vi "SLL DE Get the order of Virtual Channels.vi"(8 "error in (no error)":errorcluster, 9 "Virtial Channels Info":string[](array[string]), 10 "Number of elements":i32[](array[numeric]), 11 "Channel Names":string[][](array[string])) -> (0 "error out":errorcluster, 3 "Channel Order":i32[](array[numeric]))   [LabVIEW 2013]
doc: "Copyright © 2005, Soliton Technologies.\nAll rights reserved."
uses:
  Instance           1 48Saved   SLL DE Get the order of Virtual Channels .vi
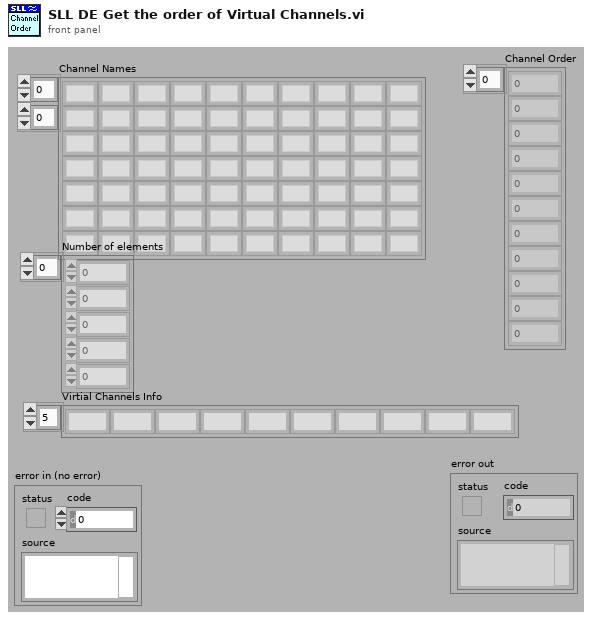
[diagram p1: front panel]
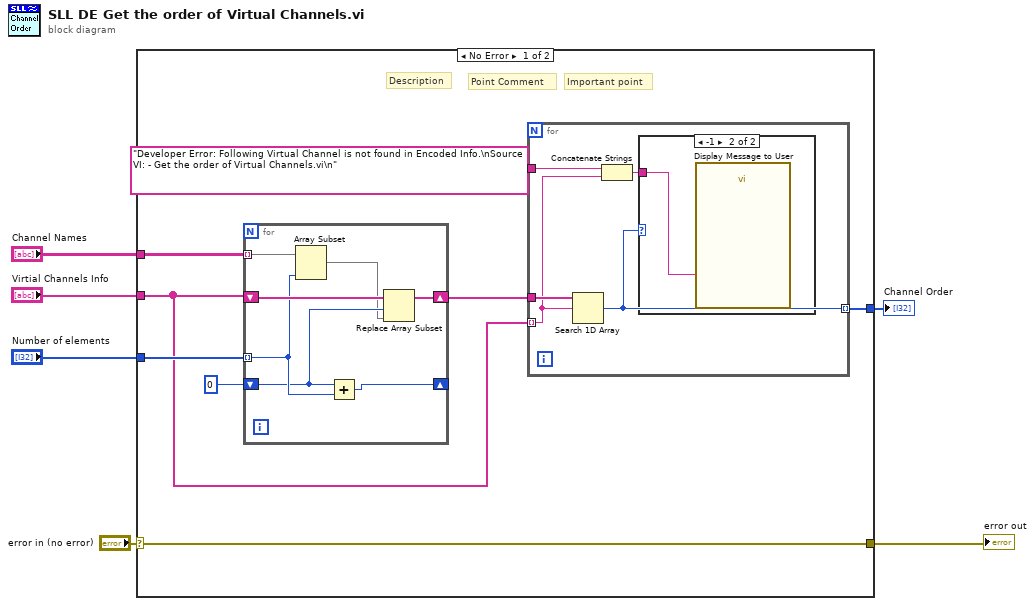
[diagram p0: block diagram]
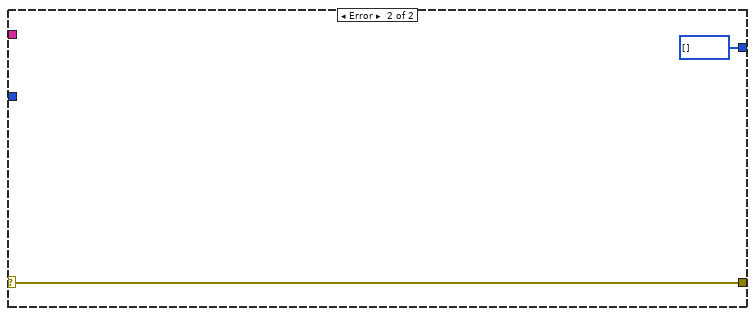
[diagram p3: hidden frame]
diagram:
  n1 = case shown="No Error" "error in (no error)" {
    selector: "error in (no error)" -> [w14 w29]
    tunnel: [w14 w29] -> w5
    tunnel: "Virtial Channels Info" -> [w9 _]
    tunnel: "Channel Names" -> [w13 _]
    tunnel: "Number of elements" -> [w12 _]
    tunnel: [w7 i32[] []] -> w1
    frame No Error {
      # "Point Comment"
      # "Important point"
      # "Description"
      n2 = for {
        tunnel: w13 -> [w27] mode=indexing
        shift-right: [w21] -> w10
        shift-left: w9 -> [w26]
        tunnel: w12 -> [w25] mode=indexing
        shift-right: [w23] -> _
        shift-left: 0 ("Virtual Channel Name") -> [w24]
        n3 = Array Subset(array=w27, length=w25) -> (w22:string[])  [unwired: 1 in]
        n4 = Add(x=w24, y=w25) -> (x+y=w23:i32)
        n5 = Replace Array Subset(array=w26, new element=w22, index=w24) -> (w21:string[])
      }
      n6 = for {
        tunnel: w10 -> [w19]
        tunnel: w9 -> [w16] mode=indexing
        tunnel: [w18] -> w7 mode=indexing
        tunnel: "Developer Error: Following Virtual Channel is not found in Encoded Info.\nSource VI: - Get the order of Virtual Channels.vi\n" ("Virtual Channel Name") -> [w17]
        n7 = Search 1D Array(1D array=w19, element=w16) -> (index of element=w18:i32)  [unwired: 1 in]
        n8 = Concatenate Strings(w17, w16) -> (w15:string)
        n9 = case shown="-1" w18 {
          tunnel: w15 -> [_ w20]
          frame 0, Default {
          }
          frame -1 {
            n10 = call "Display Message to User"("Message"=w20) -> ()  [unwired: 9 in, 2 out]
          }
        }
      }
    }
    frame Error {
    }
  }
  "error out" <- w5
  "Channel Order" <- w1
